vi "Phase_Av_Weighted_Cross_Moments.vi"(0 "AI Cluster 1":T4={"Colour"=0, "Inst type"=enum."Pitot-static tube", "Inst name"="Manometer voltage", "Symbol"="U", "Code name"="", "Extra Info"="U", "Inst Array"=enum."PWA", "Extra Titles"=[], "Extra Values"=[], "U"=0.0, "u^2"=0.0, "u^3"=0.0, "u^4"=0.0, "Skew_u"=0.0, "Kurt_u"=0.0, "Sd Error in Mean"=0.0, "% u'/U"=0.0, "X"=0.0, "Y"=0.0, "Z"=0.0, "Timescale integral Estimate"=0.0, "Sd Error in Variance"=0.0, "Calib File"=path "", "Calib Constants"=[], "Output Position"=FALSE, "Stats"=enum."None", "Av Sampling Rate"=0.0, "Av No of Samples"=0.0, "Total Meas Time (s)"=0.0, "ADAM Ch Name"="", "Max value"=0.0, "Min value"=0.0, "Req Sample Rate Hz"=0.0, "Sync Delay Time (s)"=0.0, "Ch No"=0, "Device"="", "Use Latest Calib"=FALSE, "Port"="", "Metadata Ch Names"=[], "Metadata Ch Values"=[], "Label"=""} {"Sync Delay Time (s)" format="%.4f"; "Total Meas Time (s)" format="%_5g"; "Sd Error in Variance" format="%_3g"; "Skew_u" format="%_3g"; "% u'/U" format="%_3g"; "Sd Error in Mean" format="%_3g"; "Kurt_u" format="%_3g"; "u^4" format="%_3g"; "u^3" format="%_3g"; "U" format="%_3g"; "u^2" format="%_3g"}, 1 "WT Revolution Start times":dbl[](array[numeric]), 2 "interp. method":i32(ring) items=["nearest", "linear", "spline", "cubic Hermite", "Lagrange"], 5 "Time Cluster 1":T3, 7 "AI Cluster 2":T4={"Colour"=0, "Inst type"=enum."Pitot-static tube", "Inst name"="Manometer voltage", "Symbol"="U", "Code name"="", "Extra Info"="U", "Inst Array"=enum."PWA", "Extra Titles"=[], "Extra Values"=[], "U"=0.0, "u^2"=0.0, "u^3"=0.0, "u^4"=0.0, "Skew_u"=0.0, "Kurt_u"=0.0, "Sd Error in Mean"=0.0, "% u'/U"=0.0, "X"=0.0, "Y"=0.0, "Z"=0.0, "Timescale integral Estimate"=0.0, "Sd Error in Variance"=0.0, "Calib File"=path "", "Calib Constants"=[], "Output Position"=FALSE, "Stats"=enum."None", "Av Sampling Rate"=0.0, "Av No of Samples"=0.0, "Total Meas Time (s)"=0.0, "ADAM Ch Name"="", "Max value"=0.0, "Min value"=0.0, "Req Sample Rate Hz"=0.0, "Sync Delay Time (s)"=0.0, "Ch No"=0, "Device"="", "Use Latest Calib"=FALSE, "Port"="", "Metadata Ch Names"=[], "Metadata Ch Values"=[], "Label"=""} {"Sync Delay Time (s)" format="%.4f"; "Total Meas Time (s)" format="%_5g"; "Sd Error in Variance" format="%_3g"; "Skew_u" format="%_3g"; "% u'/U" format="%_3g"; "Sd Error in Mean" format="%_3g"; "Kurt_u" format="%_3g"; "u^4" format="%_3g"; "u^3" format="%_3g"; "U" format="%_3g"; "u^2" format="%_3g"}, 9 "Time Cluster 2":T3, 11 "Shift In":T1[](array[typedef]), 12 "Shift Cluster In":T2[](array[typedef]) {"Cross Correlation" format="%.2f"; "Stats" format="%.2f"}, 13 "No Of Bins":i32) -> (4 "Phase locked uw":dbl[](array[numeric]), 6 "Phase locked uw/u'w'":dbl[](array[numeric]), 14 "Shift Cluster Out":T2[](array[typedef]) {"Cross Correlation" format="%.2f"; "Stats" format="%.2f"}, 15 "Shift Out":T1[](array[typedef]))   [LabVIEW 2021]
uses:
  Globals/Meas_global.vi
  Controls/Inst_type.ctl
  Controls/Instrument_Array.ctl
  Controls/Analysis_info_cluster.ctl
  Controls/Time_Trace_Cluster.ctl
  Controls/Cross_Moments_Shift_Cluster.ctl
  Controls/Shift_Cluster.ctl
panel:
  out "Array":cluster{"Points":dbl[][]}[](array[cluster])
  in  "Time Cluster 3":cluster{"Points":dbl[][]}
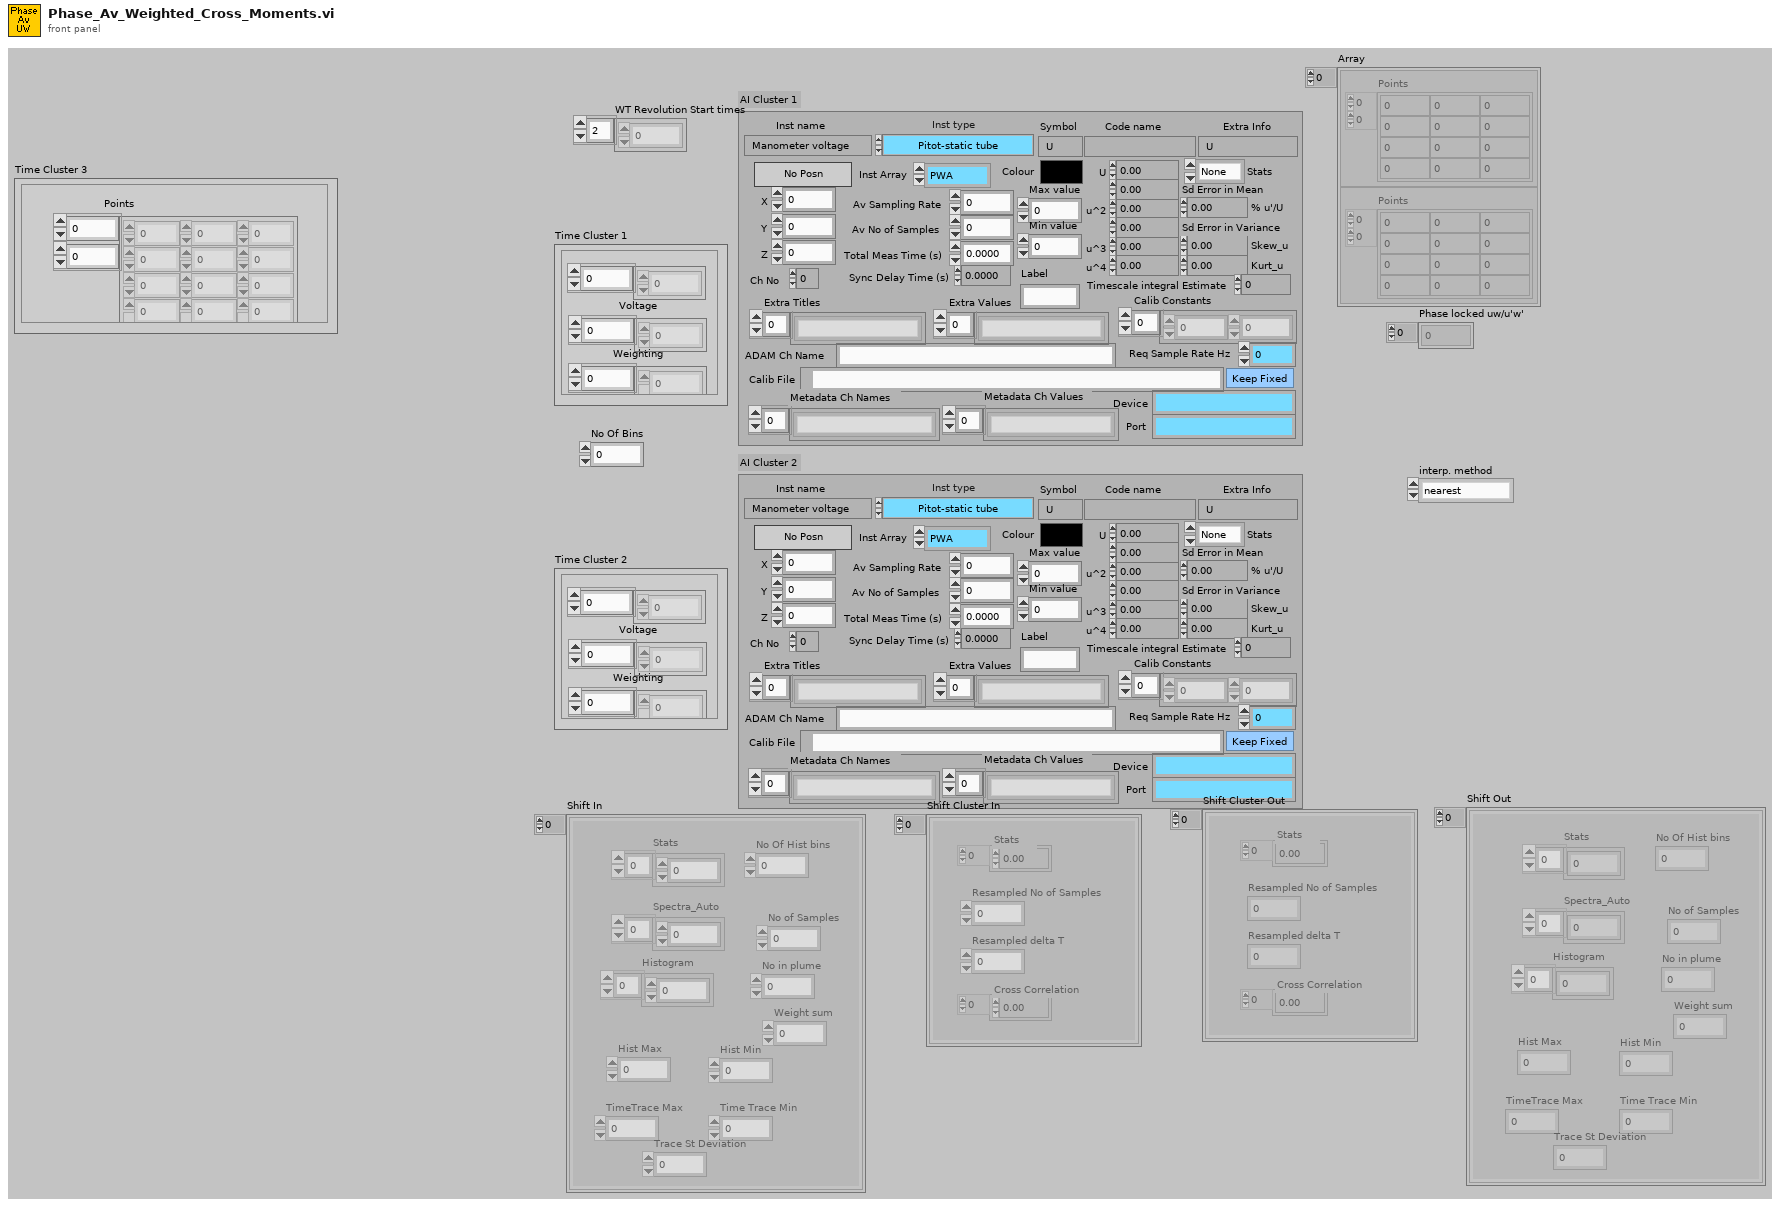
[diagram p1: front panel]
types:
  T1 = typedef "Shift_Cluster.ctl" = cluster{"Stats":dbl[], "Spectra_Auto":dbl[], "Histogram":dbl[], "Hist Max":dbl, "Hist Min":dbl, "No of Samples":i32, "No in plume":i32, "Weight sum":dbl, "No Of Hist bins":i32, "TimeTrace Max":dbl, "Time Trace Min":dbl, "Trace St Deviation":dbl}
  T2 = typedef "Cross_Moments_Shift_Cluster.ctl" = cluster{"Stats":dbl[], "Resampled No of Samples":i32, "Resampled delta T":dbl, "Cross Correlation":dbl[]}
  T3 = typedef "Time_Trace_Cluster.ctl" = cluster{"Weighting":dbl[], "Voltage":dbl[], "Eng Values":dbl[]}
  T4 = typedef "Analysis_info_cluster.ctl" = cluster{"Colour":u32, "Inst type":T5, "Inst name":string, "Symbol":string, "Code name":string, "Extra Info":string, "Inst Array":T6, "Extra Titles":string[], "Extra Values":string[], "U":dbl, "u^2":dbl, "u^3":dbl, "u^4":dbl, "Skew_u":dbl, "Kurt_u":dbl, "Sd Error in Mean":dbl, "% u'/U":dbl, "X":dbl, "Y":dbl, "Z":dbl, "Timescale integral Estimate":dbl, "Sd Error in Variance":dbl, "Calib File":path, "Calib Constants":dbl[], "Output Position":bool, "Stats":enum16{"None", "Basic", "Full"}, "Av Sampling Rate":dbl, "Av No of Samples":dbl, "Total Meas Time (s)":dbl, "ADAM Ch Name":string, "Max value":dbl, "Min value":dbl, "Req Sample Rate Hz":dbl, "Sync Delay Time (s)":dbl, "Ch No":i16, "Device":string, "Use Latest Calib":bool, "Port":string, "Metadata Ch Names":string[], "Metadata Ch Values":string[], "Label":string}
  T5 = typedef "Inst_type.ctl" = enum16{"Raw voltage", "Raw with zero offsetting", "Propeller anemometer", "Pressure Transducer", "Pitot-static tube", "Hot wire", "Cross wire 1", "Cross wire 2", "Generic Linear", "Generic Polynomial", "Generic BackPoly", "Fast FID", "Thermocouple", "Cold wire", "Pulsed Wire", "LDA Vel", "LDA Tran time", "LDA Arr time", "Microphone"}
  T6 = typedef "Instrument_Array.ctl" = enum16{"PWA", "LDA", "Analogue"}
  T7 = typedef "Correlation_cluster1.ctl" = cluster{"U inst":string, "uw":dbl, "u^2w":dbl, "uw^2":dbl, "uw/u'w'":dbl, "W inst":string, "uw^3":dbl, "u^3w":dbl, "u^2w^2":dbl, "Index U":i32, "Index W":i32, "Error info":string[], "Paired Sampling Rate (Hz)":dbl, "u^2 Paired":dbl, "w^2 Paired":dbl, "Time Window (ms)":dbl}
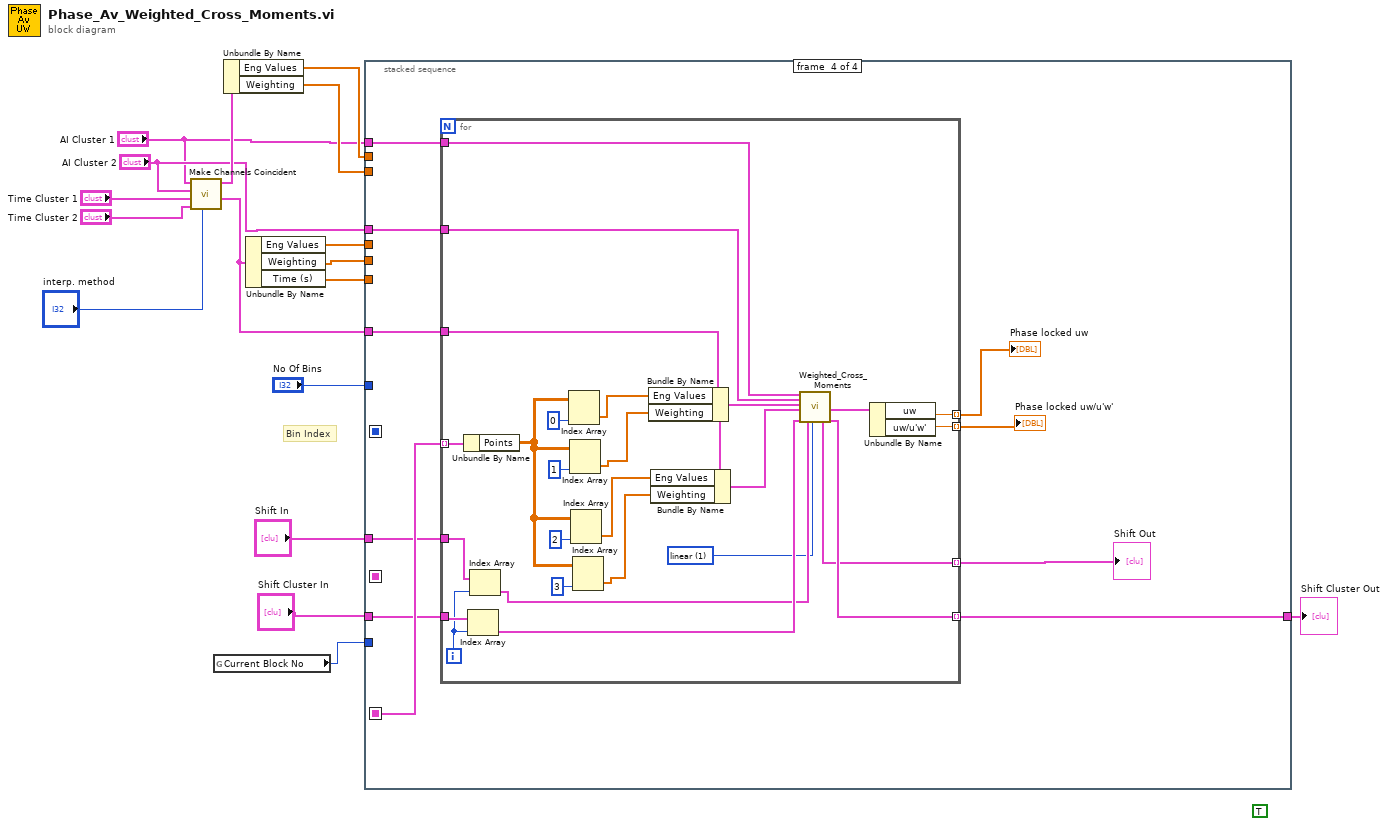
[diagram p0: block diagram]
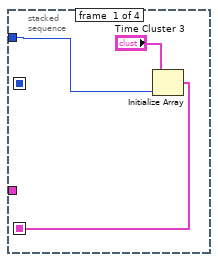
[diagram p2: hidden frame]
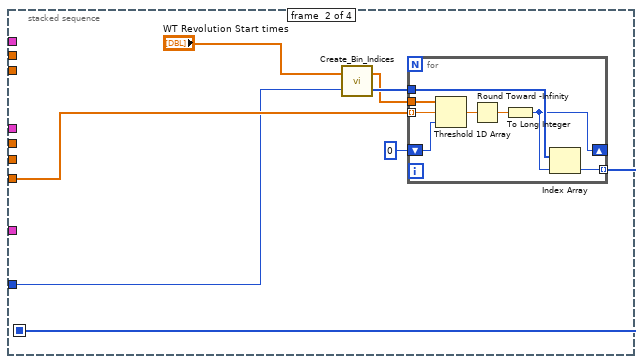
[diagram p3: hidden frame]
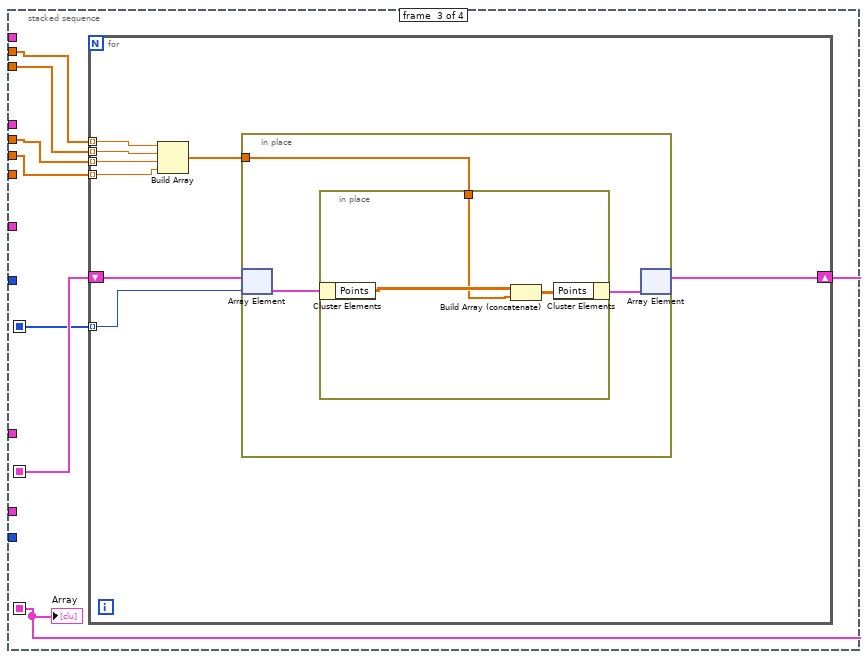
[diagram p4: hidden frame]
diagram:
  (unwired) TRUE
  # "Bin Index"
  n1 = call "Make Channels Coincident.vi"("interp. method"="interp. method", "Time Cluster 2"="Time Cluster 2", "Time Cluster 1"="Time Cluster 1", "Cluster 2"="AI Cluster 2", "Cluster 1"="AI Cluster 1") -> ("Coincident Time Cluster 2"=w8:T3, "Coincident Time Cluster 1"=w9:T3)  [unwired: 4 in, 1 out]
  n2 = global read "Meas_global.vi" "Current Block No"() -> (w17:i32)
  n3 = Unbundle By Name(w9) -> ("Eng Values"=w16:dbl[], "Weighting"=w15:dbl[])
  n4 = Unbundle By Name(w8) -> ("Eng Values"=w14:dbl[], "Weighting"=w13:dbl[], "Time (s)"=w7:dbl[])
  n5 = stacked-sequence {
    seq-local: [_ w22 _ _] -> [_ _ w41 _]
    seq-local: [w18 _ _ _] -> [_ _ w42 _]
    seq-local: [_ _ w36 _] -> [_ _ _ w65]
    tunnel: w16 -> [_ _ w40 _]
    tunnel: "Shift Cluster In" -> [_ _ _ w62]
    tunnel: w14 -> [_ _ w38 _]
    tunnel: w17 -> [_ _ _ _]
    tunnel: w15 -> [_ _ w39 _]
    tunnel: w13 -> [_ _ w37 _]
    tunnel: "AI Cluster 1" -> [_ _ _ w64]
    tunnel: "AI Cluster 2" -> [_ _ _ w63]
    tunnel: [_ _ _ w61] -> w3
    tunnel: w8 -> [_ _ _ w66]
    tunnel: w7 -> [_ w23 _ _]
    tunnel: "No Of Bins" -> [w20 w21 _ _]
    tunnel: "Shift In" -> [_ _ _ w57]
    frame #0 {
      n6 = Initialize Array("Time Cluster 3", w20) -> (w18:cluster{"Points":dbl[][]}[])
    }
    frame #1 {
      n7 = call "Create_Bin_Indices.vi"("No Of Bins"=w21, "Cycle Start TIme"="WT Revolution Start times") -> ("Bin Number"=w27:i32[], "Bin Start Time"=w26:dbl[])
      n8 = for {
        tunnel: w26 -> [w35]
        tunnel: w23 -> [w34] mode=indexing
        shift-right: [w31] -> _
        shift-left: 0 -> [w28]
        tunnel: w27 -> [w32]
        tunnel: [w30] -> w22 mode=indexing
        n9 = Threshold 1D Array(1:w28, 2:w34, 3:w35) -> (0:w33:dbl)
        n10 = Round Toward -Infinity(1:w33) -> (0:w29:dbl)
        n11 = To Long Integer(number=w29) -> (32bit integer=w31:i32)
        n12 = Index Array(array=w32, index=w31) -> (element=w30:i32)
      }
    }
    frame #2 {
      n13 = for {
        shift-right: [w48] -> w36
        shift-left: w42 -> [w49]
        tunnel: w41 -> [w50] mode=indexing
        tunnel: w40 -> [w47] mode=indexing
        tunnel: w39 -> [w46] mode=indexing
        tunnel: w38 -> [w45] mode=indexing
        tunnel: w37 -> [w44] mode=indexing
        n14 = Build Array(w47, w46, w45, w44) -> (w43:dbl[])
        n15 = in-place {
          in-place-border: w43 -> [w51]
          n16 = in-place-array #1(w49, w50) -> (w53:cluster{"Points":dbl[][]})
          n17 = in-place {
            in-place-border: w51 -> [w55]
            n18 = in-place-cluster #2(w53) -> ("Points"=w56:dbl[][])
            n19 = Build Array (concatenate)(w56, w55) -> (w54:dbl[][])
            n20 = in-place-cluster #2("Points"=w54) -> (w52:cluster{"Points":dbl[][]})
          }
          n21 = in-place-array #1(w52) -> (w48:cluster{"Points":dbl[][]}[])  [unwired: 1 out]
        }
      }
      "Array" <- w36
    }
    frame #3 {
      n22 = for {
        tunnel: w66 -> [w92]
        tunnel: w65 -> [w91] mode=indexing
        tunnel: w64 -> [w81]
        tunnel: w63 -> [w80]
        tunnel: w62 -> [w76]
        tunnel: [w77] -> w61 mode=indexing
        tunnel: [w73] -> w60 mode=indexing
        tunnel: [w72] -> w59 mode=indexing
        tunnel: [w70] -> w58 mode=indexing
        tunnel: w57 -> [w69]
        i -> [w71]
        w67 = 1 items=["nearest", "linear", "spline", "cubic Hermite", "Lagrange"] ("interp. method")
        n23 = Unbundle By Name(w91) -> ("Points"=w85:dbl[][])
        n24 = Index Array(array=w76, index=w71) -> (element=w75:T2)
        n25 = Index Array(array=w69, index=w71) -> (element=w68:T1)
        n26 = Index Array(array=w85, index (col)=0 ("disabled index (col)")) -> (element=w89:dbl[])  [unwired: 1 in]
        n27 = Index Array(array=w85, index (col)=1 ("disabled index (col)")) -> (element=w82:dbl[])  [unwired: 1 in]
        n28 = Index Array(array=w85, index (col)=2 ("disabled index (col)")) -> (element=w84:dbl[])  [unwired: 1 in]
        n29 = Index Array(array=w85, index (col)=3 ("disabled index (col)")) -> (element=w83:dbl[])  [unwired: 1 in]
        n30 = Bundle By Name(cluster=w92, "Eng Values"=w89, "Weighting"=w82) -> (w79:T3)
        n31 = Bundle By Name(cluster=w92, "Eng Values"=w84, "Weighting"=w83) -> (w78:T3)
        n32 = call "Weighted_Cross_Moments.vi"("AI Cluster 1"=w81, "AI Cluster 2"=w80, "Time Cluster 1"=w79, "Time Cluster 2"=w78, "Shift Cluster In"=w75, "Shift Input"=w68, "interp. method"=w67) -> ("Shift Output"=w70:T1, "output cluster"=w74:T7, "Shift Cluster Out"=w77:T2)  [unwired: 10 in]
        n33 = Unbundle By Name(w74) -> ("uw"=w73:dbl, "uw/u'w'"=w72:dbl)
      }
      "Phase locked uw" <- w60
      "Phase locked uw/u'w'" <- w59
      "Shift Out" <- w58
    }
  }
  "Shift Cluster Out" <- w3
